vi "AUTON_Index.vi"(0 "Auton Array":dbl[][](array[numeric]), 5 "MeasuredHeading":dbl, 7 "LeftEncoder":dbl, 9 "RightEncoder":dbl) -> (4 "Left Drive":dbl, 6 "Right Drive":dbl, 8 "Indexer":dbl, 10 "Shooter Elevation":dbl, 13 "Flipper":dbl, 14 "Roller":dbl, 15 "Shooter Wheels":dbl)   [LabVIEW 2012]
uses:
  Robot Global Data.vi
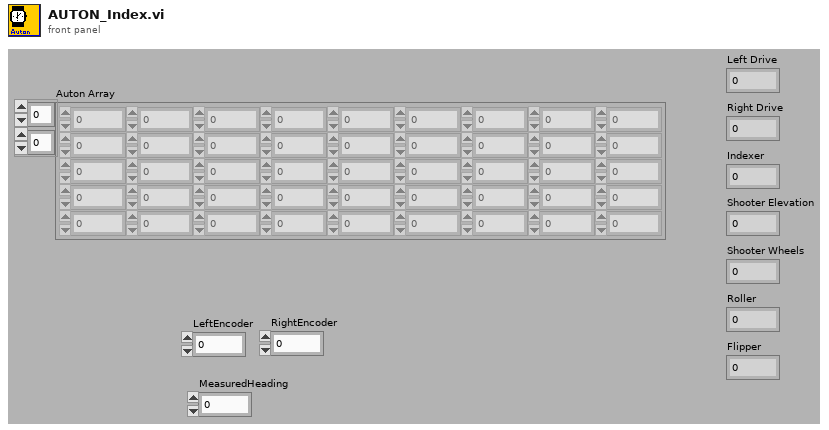
[diagram p1: front panel]
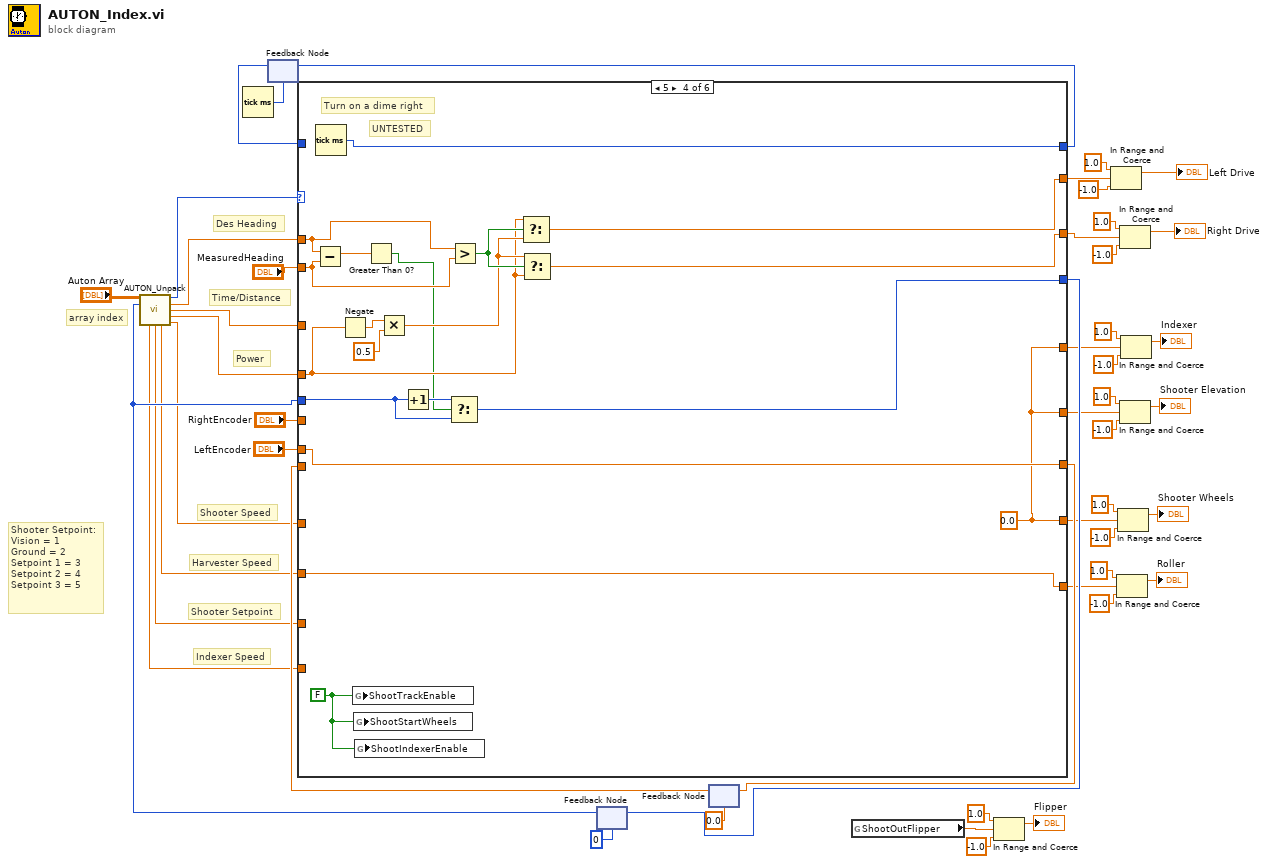
[diagram p0: block diagram]
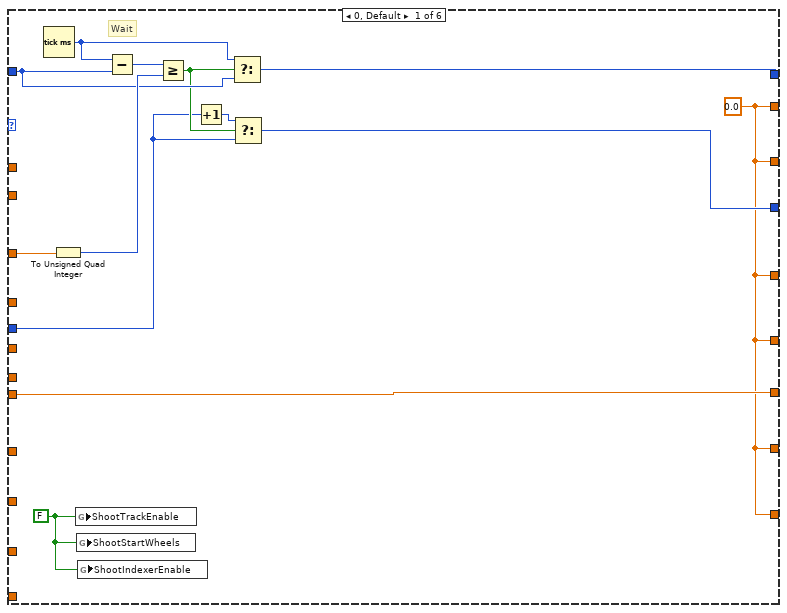
[diagram p2: hidden frame]
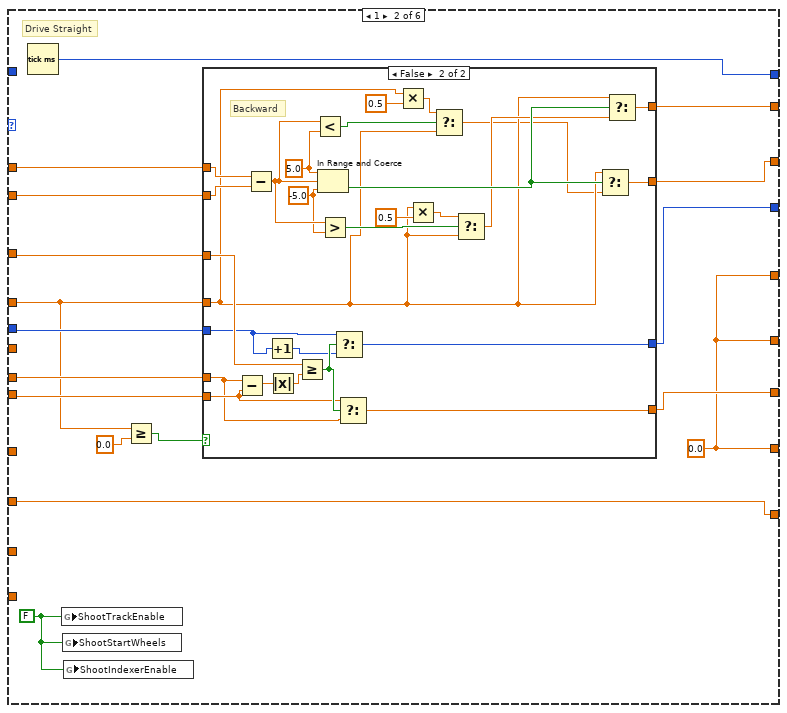
[diagram p3: hidden frame]
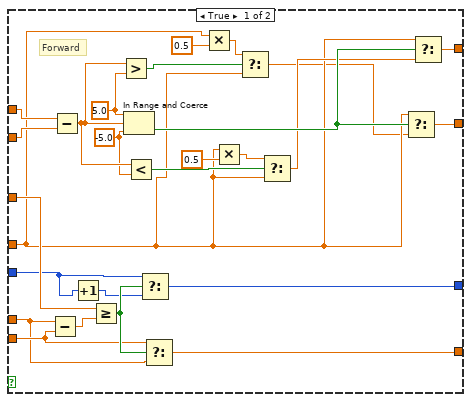
[diagram p4: hidden frame]
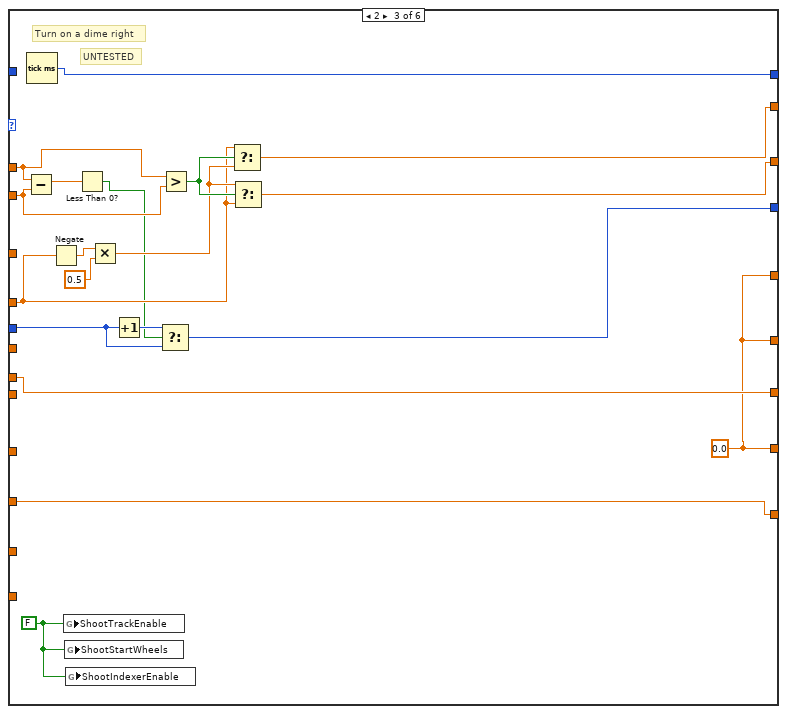
[diagram p5: hidden frame]
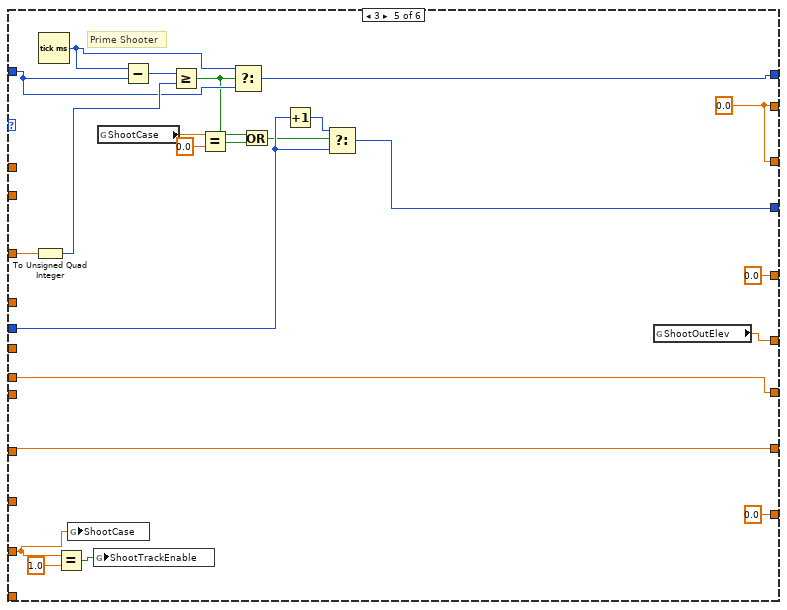
[diagram p6: hidden frame]
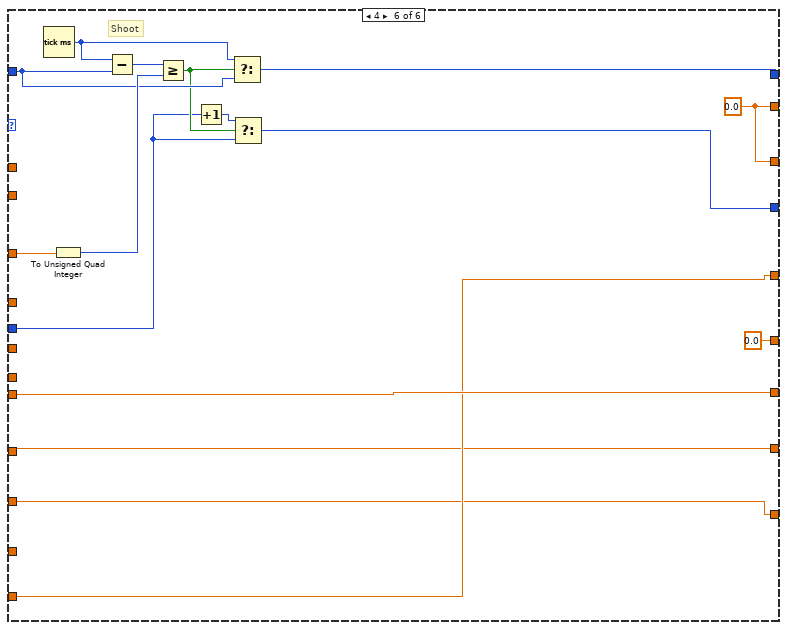
[diagram p7: hidden frame]
diagram:
  # "Shooter Setpoint:\nVision = 1\nGround = 2\nSetpoint 1 = 3\nSetpoint 2 = 4\nSetpoint 3 = 5"
  # "Indexer Speed"
  # "Shooter Speed"
  # "Shooter Setpoint"
  # "Harvester Speed"
  # "Des Heading"
  # "Time/Distance"
  # "Power"
  # "array index"
  n1 = Tick Count (ms)() -> (millisecond timer value=w46:u32)
  n2 = feedback #1(w46) -> (w48:u32)
  n3 = feedback #2(0) -> (w25:i32)
  n4 = call "AUTON_Unpack.vi"("all rows"="Auton Array", "Index"=w25) -> ("Primitive ID"=w29:i16, "Desired Heading"=w27:dbl, "Time/Distance"=w26:dbl, "Power"=w28:dbl, "Indexer Speed"=w21:dbl, "Shooter Setpoint"=w22:dbl, "Harvester Speed"=w23:dbl, "Shooter Speed"=w24:dbl)  [unwired: 6 in]
  n5 = feedback #3(0.0) -> (w31:dbl)
  n6 = case shown="5" w29 {
    tunnel: [w54 w77 w146 w165 w185 w201] -> w34
    tunnel: w25 -> [w55 w72 w149 w168 w176 w202]
    tunnel: [w62 w69 w151 w170 w174 w209] -> w36
    tunnel: w48 -> [w59 _ _ _ w175 w206]
    tunnel: w26 -> [w53 w78 _ _ w177 w200]
    tunnel: w27 -> [_ w76 w144 w163 _ _]
    tunnel: [w51 w74 w147 w166 w193 w198] -> w44
    tunnel: [w51 w73 w148 w167 w193 w198] -> w37
    tunnel: w28 -> [_ w68 w138 w157 _ _]
    tunnel: "LeftEncoder" -> [_ w70 w145 w164 w192 _]
    tunnel: "MeasuredHeading" -> [_ w75 w143 w162 _ _]
    tunnel: "RightEncoder" -> [_ _ _ _ _ _]
    tunnel: w31 -> [w52 w71 _ _ _ w199]
    tunnel: [w52 w79 w145 w164 w192 w199] -> w30
    tunnel: w24 -> [_ _ _ _ w191 w195]
    tunnel: w23 -> [_ w63 w135 w154 _ w194]
    tunnel: w22 -> [_ _ _ _ w181 _]
    tunnel: w21 -> [_ _ _ _ _ w197]
    tunnel: [w51 w63 w135 w154 0.0 ("Harvester Speed") w194] -> w5
    tunnel: [w51 w65 w136 w155 w191 w195] -> w4
    tunnel: [w51 w65 w136 w155 w188 0.0 ("ShootOutElev")] -> w3
    tunnel: [w51 w65 w136 w155 0.0 ("Numeric") w197] -> w2
    frame 0, Default {
      w50 = FALSE ("ShootTrackEnable")
      w51 = 0.0 ("Numeric")
      # "Wait"
      n7 = Tick Count (ms)() -> (millisecond timer value=w58:u32)
      n8 = To Unsigned Quad Integer(1:w53) -> (0:w60:u64)
      n9 = global write "Robot Global Data.vi" "ShootTrackEnable"(w50) -> ()
      n10 = global write "Robot Global Data.vi" "ShootStartWheels"(w50) -> ()
      n11 = global write "Robot Global Data.vi" "ShootIndexerEnable"(w50) -> ()
      n12 = Subtract(x=w58, y=w59) -> (x-y=w61:u32)
      n13 = Greater Or Equal?(x=w61, y=w60) -> (x >= y?=w57:bool)
      n14 = Increment(x=w55) -> (x+1=w56:i32)
      n15 = Select(t=w58, s=w57, f=w59) -> (s? t:f=w62:u32)
      n16 = Select(t=w56, s=w57, f=w55) -> (s? t:f=w54:i32)
    }
    frame 1 {
      w64 = FALSE ("ShootTrackEnable")
      w65 = 0.0 ("Numeric")
      # "Drive Straight"
      n17 = Tick Count (ms)() -> (millisecond timer value=w69:u32)
      n18 = global write "Robot Global Data.vi" "ShootTrackEnable"(w64) -> ()
      n19 = global write "Robot Global Data.vi" "ShootStartWheels"(w64) -> ()
      n20 = global write "Robot Global Data.vi" "ShootIndexerEnable"(w64) -> ()
      n21 = Greater Or Equal?(x=w68, y=0.0) -> (x >= y?=w66:bool)
      n22 = case shown="False" w66 {
        tunnel: [w105 w132] -> w79
        tunnel: w78 -> [w103 w131]
        tunnel: [w101 w129] -> w77
        tunnel: w76 -> [w100 w128]
        tunnel: w75 -> [w99 w127]
        tunnel: [w97 w125] -> w74
        tunnel: [w96 w124] -> w73
        tunnel: w68 -> [w85 w113]
        tunnel: w72 -> [w82 w110]
        tunnel: w71 -> [w81 w109]
        tunnel: w70 -> [w80 w108]
        frame True {
          w93 = -5.0 ("lower limit")
          w95 = 5.0 ("upper limit")
          # "Forward"
          n23 = Subtract(x=w80, y=w81) -> (x-y=w104:dbl)
          n24 = Subtract(x=w100, y=w99) -> (x-y=w94:dbl)
          n25 = Increment(x=w82) -> (x+1=w83:i32)
          n26 = Greater Or Equal?(x=w103, y=w104) -> (x >= y?=w102:bool)
          n27 = Greater?(x=w94, y=w95) -> (0:w88:bool)
          n28 = In Range and Coerce(upper limit=w95, x=w94, lower limit=w93) -> (In Range?=w98:bool)  [unwired: 1 out]
          n29 = Less?(x=w94, y=w93) -> (x < y?=w92:bool)
          n30 = Select(t=w82, s=w102, f=w83) -> (s? t:f=w101:i32)
          n31 = Select(t=w81, s=w102, f=w80) -> (s? t:f=w105:dbl)
          n32 = Multiply(x=w85, y=0.5) -> (x*y=w87:dbl)
          n33 = Multiply(x=w85, y=0.5) -> (x*y=w90:dbl)
          n34 = Select(t=w87, s=w88, f=w85) -> (s? t:f=w84:dbl)
          n35 = Select(t=w90, s=w92, f=w85) -> (s? t:f=w89:dbl)
          n36 = Select(t=w85, s=w98, f=w84) -> (s? t:f=w96:dbl)
          n37 = Select(t=w85, s=w98, f=w89) -> (s? t:f=w97:dbl)
        }
        frame False {
          w121 = -5.0 ("lower limit")
          w123 = 5.0 ("upper limit")
          # "Backward"
          n38 = Subtract(x=w108, y=w109) -> (x-y=w106:dbl)
          n39 = Subtract(x=w128, y=w127) -> (x-y=w122:dbl)
          n40 = Increment(x=w110) -> (x+1=w111:i32)
          n41 = Absolute Value(x=w106) -> (abs(x)=w107:dbl)
          n42 = Greater Or Equal?(x=w131, y=w107) -> (x >= y?=w130:bool)
          n43 = Less?(x=w122, y=w123) -> (x < y?=w116:bool)
          n44 = In Range and Coerce(upper limit=w123, x=w122, lower limit=w121) -> (In Range?=w126:bool)  [unwired: 1 out]
          n45 = Greater?(x=w122, y=w121) -> (0:w120:bool)
          n46 = Select(t=w110, s=w130, f=w111) -> (s? t:f=w129:i32)
          n47 = Select(t=w109, s=w130, f=w108) -> (s? t:f=w132:dbl)
          n48 = Multiply(x=w113, y=0.5) -> (x*y=w115:dbl)
          n49 = Multiply(x=w113, y=0.5) -> (x*y=w118:dbl)
          n50 = Select(t=w115, s=w116, f=w113) -> (s? t:f=w112:dbl)
          n51 = Select(t=w118, s=w120, f=w113) -> (s? t:f=w117:dbl)
          n52 = Select(t=w113, s=w126, f=w112) -> (s? t:f=w124:dbl)
          n53 = Select(t=w113, s=w126, f=w117) -> (s? t:f=w125:dbl)
        }
      }
    }
    frame 2 {
      w136 = 0.0 ("Numeric")
      w137 = FALSE ("ShootTrackEnable")
      # "UNTESTED"
      # "Turn on a dime right"
      n54 = Subtract(x=w144, y=w143) -> (x-y=w134:dbl)
      n55 = Tick Count (ms)() -> (millisecond timer value=w151:u32)
      n56 = Negate(x=w138) -> (-x=w141:dbl)
      n57 = global write "Robot Global Data.vi" "ShootTrackEnable"(w137) -> ()
      n58 = global write "Robot Global Data.vi" "ShootStartWheels"(w137) -> ()
      n59 = global write "Robot Global Data.vi" "ShootIndexerEnable"(w137) -> ()
      n60 = Less Than 0?(x=w134) -> (x < 0?=w133:bool)
      n61 = Multiply(x=w141, y=0.5) -> (x*y=w139:dbl)
      n62 = Increment(x=w149) -> (x+1=w150:i32)
      n63 = Select(t=w150, s=w133, f=w149) -> (s? t:f=w146:i32)
      n64 = Greater?(x=w144, y=w143) -> (0:w142:bool)
      n65 = Select(t=w138, s=w142, f=w139) -> (s? t:f=w147:dbl)
      n66 = Select(t=w139, s=w142, f=w138) -> (s? t:f=w148:dbl)
    }
    frame 5 {
      w155 = 0.0 ("Numeric")
      w156 = FALSE ("ShootTrackEnable")
      # "UNTESTED"
      # "Turn on a dime right"
      n67 = Subtract(x=w163, y=w162) -> (x-y=w153:dbl)
      n68 = Tick Count (ms)() -> (millisecond timer value=w170:u32)
      n69 = Negate(x=w157) -> (-x=w160:dbl)
      n70 = global write "Robot Global Data.vi" "ShootTrackEnable"(w156) -> ()
      n71 = global write "Robot Global Data.vi" "ShootStartWheels"(w156) -> ()
      n72 = global write "Robot Global Data.vi" "ShootIndexerEnable"(w156) -> ()
      n73 = Greater Than 0?(x=w153) -> (x > 0?=w152:bool)
      n74 = Multiply(x=w160, y=0.5) -> (x*y=w158:dbl)
      n75 = Increment(x=w168) -> (x+1=w169:i32)
      n76 = Select(t=w169, s=w152, f=w168) -> (s? t:f=w165:i32)
      n77 = Greater?(x=w163, y=w162) -> (0:w161:bool)
      n78 = Select(t=w157, s=w161, f=w158) -> (s? t:f=w166:dbl)
      n79 = Select(t=w158, s=w161, f=w157) -> (s? t:f=w167:dbl)
    }
    frame 3 {
      w193 = 0.0 ("Power")
      # "Prime Shooter"
      n80 = To Unsigned Quad Integer(1:w177) -> (0:w179:u64)
      n81 = Tick Count (ms)() -> (millisecond timer value=w178:u32)
      n82 = Equal?(x=w181, y=1.0) -> (x = y?=w182:bool)
      n83 = global write "Robot Global Data.vi" "ShootCase"(w181) -> ()
      n84 = global write "Robot Global Data.vi" "ShootTrackEnable"(w182) -> ()
      n85 = global read "Robot Global Data.vi" "ShootCase"() -> (w187:dbl)
      n86 = Subtract(x=w178, y=w175) -> (x-y=w180:u32)
      n87 = Greater Or Equal?(x=w180, y=w179) -> (x >= y?=w171:bool)
      n88 = Equal?(x=w187, y=0.0) -> (x = y?=w173:bool)
      n89 = Select(t=w178, s=w171, f=w175) -> (s? t:f=w174:u32)
      n90 = Or(x=w171, y=w173) -> (x .or. y?=w172:bool)
      n91 = Increment(x=w176) -> (x+1=w184:i32)
      n92 = Select(t=w184, s=w172, f=w176) -> (s? t:f=w185:i32)
      n93 = global read "Robot Global Data.vi" "ShootOutElev"() -> (w188:dbl)
    }
    frame 4 {
      w198 = 0.0 ("Numeric")
      # "Shoot"
      n94 = Tick Count (ms)() -> (millisecond timer value=w205:u32)
      n95 = To Unsigned Quad Integer(1:w200) -> (0:w207:u64)
      n96 = Subtract(x=w205, y=w206) -> (x-y=w208:u32)
      n97 = Greater Or Equal?(x=w208, y=w207) -> (x >= y?=w204:bool)
      n98 = Increment(x=w202) -> (x+1=w203:i32)
      n99 = Select(t=w205, s=w204, f=w206) -> (s? t:f=w209:u32)
      n100 = Select(t=w203, s=w204, f=w202) -> (s? t:f=w201:i32)
    }
  }
  n101 = feedback-in #1(w36) -> ()
  n102 = feedback-in #2(w34) -> ()
  n103 = feedback-in #3(w30) -> ()
  n104 = global read "Robot Global Data.vi" "ShootOutFlipper"() -> (w1:dbl)
  n105 = In Range and Coerce(upper limit=1.0, x=w1, lower limit=-1.0) -> (coerced(x)=→"Flipper":dbl)  [unwired: 1 out]
  n106 = In Range and Coerce(upper limit=1.0, x=w44, lower limit=-1.0) -> (coerced(x)=→"Left Drive":dbl)  [unwired: 1 out]
  n107 = In Range and Coerce(upper limit=1.0, x=w5, lower limit=-1.0) -> (coerced(x)=→"Roller":dbl)  [unwired: 1 out]
  n108 = In Range and Coerce(upper limit=1.0, x=w4, lower limit=-1.0) -> (coerced(x)=→"Shooter Wheels":dbl)  [unwired: 1 out]
  n109 = In Range and Coerce(upper limit=1.0, x=w37, lower limit=-1.0) -> (coerced(x)=→"Right Drive":dbl)  [unwired: 1 out]
  n110 = In Range and Coerce(upper limit=1.0, x=w3, lower limit=-1.0) -> (coerced(x)=→"Shooter Elevation":dbl)  [unwired: 1 out]
  n111 = In Range and Coerce(upper limit=1.0, x=w2, lower limit=-1.0) -> (coerced(x)=→"Indexer":dbl)  [unwired: 1 out]
